vi "runner.vi"() -> ()   [LabVIEW 2010]
uses:
  common/xcontrols/XUserDropdown/XUserDropdown/XUserDropdown.xctl
  common/classes/ErrorController/ErrorController/ErrorController.lvclass
  <vilib>/Utility/miscctls.llb/LVPointTypeDef.ctl
  common/clusters/plugin_specification.ctl
  HelioWizardDL101109/wizard_cluster.ctl
  common/classes/GenericComponent/GenericComponent/GenericComponent.lvclass
  <vilib>/Platform/browser.llb/Open URL in Default Browser (string).vi
  common/classes/ErrorController/ErrorController/class_data.vi
panel:
  out "error loaded?":bool
  out "progress slider":i32(slide) scale=0.0..17.0
  in  "button: copy user":bool
  in  "button: delete user":bool
  in  "button: new user":bool
  in  "user":string(xcontrol)
  in  "mainConfigButton":bool
  in  "step":i32(listbox) caption="steps"
  in  "proceedButton":bool
  in  "backButton":bool
  in  "startButton":bool
  in  "wizard":string(combo) caption="Select a wizard"
  # "Wizard Runner"
  # "Procedure\n\n1. Select and start a wizard (it may take some time until all steps are loaded).\n\n2. Perform all configuration steps in the sequence given (note that there may be dependencies!).\n\n3. Edit main configuration.\n\nHint: Don't leave any component specifications empty in the configuration dialogs. Choose the generic version if a more specifiy component doesn't apply."
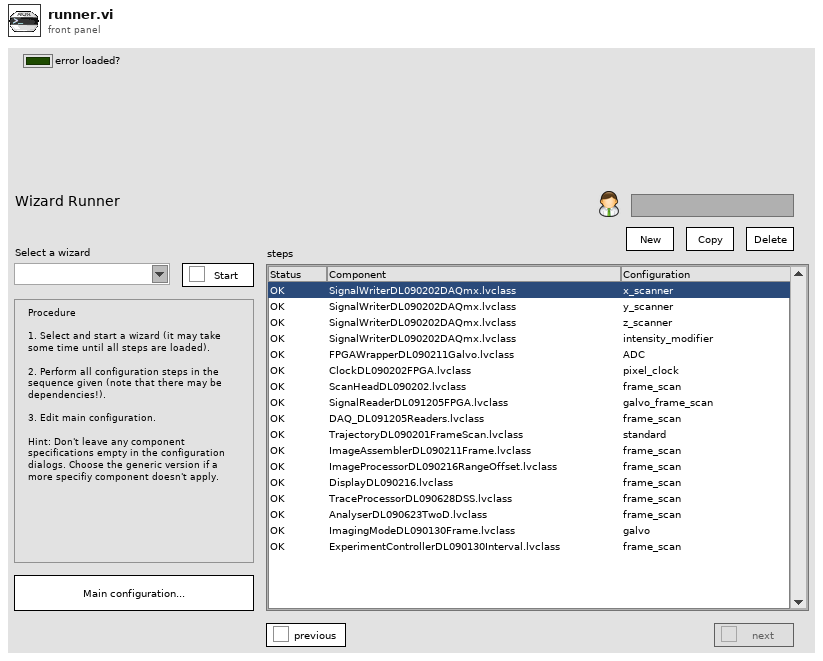
[diagram p1: front panel]
types:
  T1 = typedef "LVPointTypeDef.ctl" = cluster{"Horizontal":i16, "Vertical":i16}
  T2 = typedef "plugin_specification.ctl" = cluster{"class path":string, "configuration":string, "label":string, "settings name":string}
  T3 = typedef "wizard_cluster.ctl" = cluster{"step":T2[]}
  T4 = enum8{"Enabled", "Disabled", "Disabled and Grayed Out"}
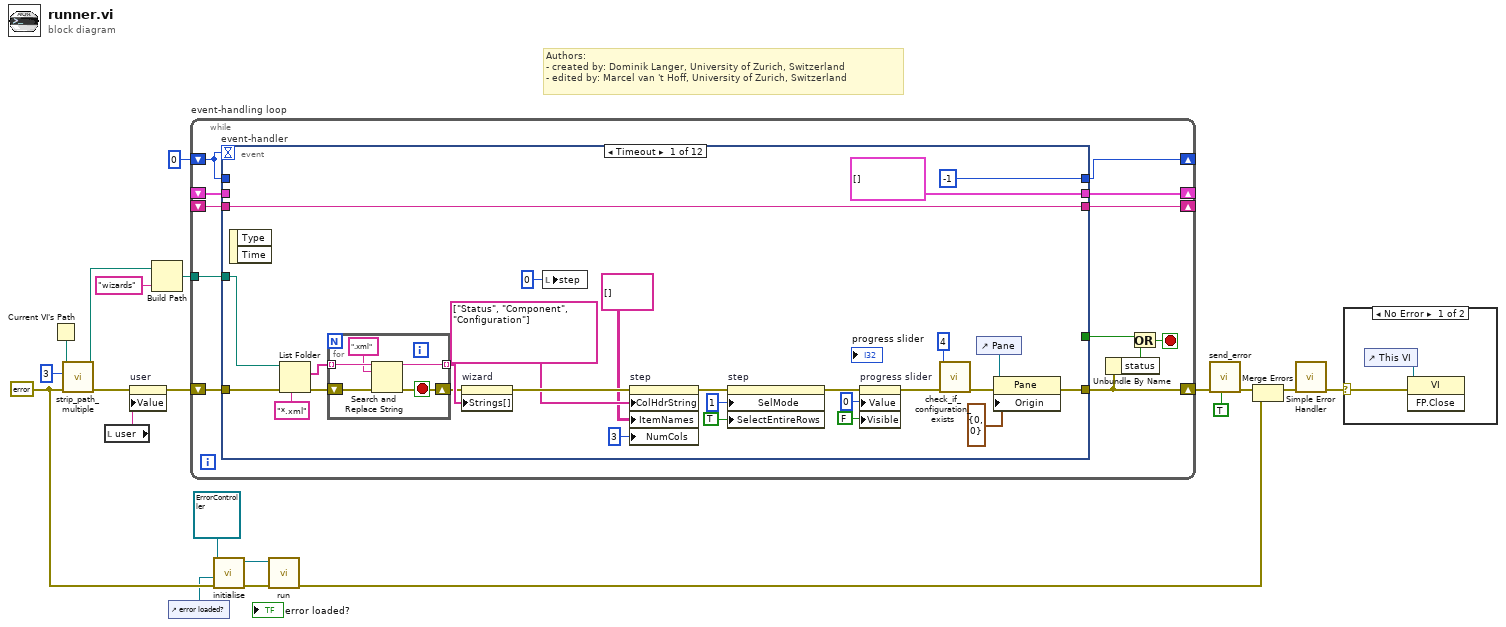
[diagram p0: block diagram]
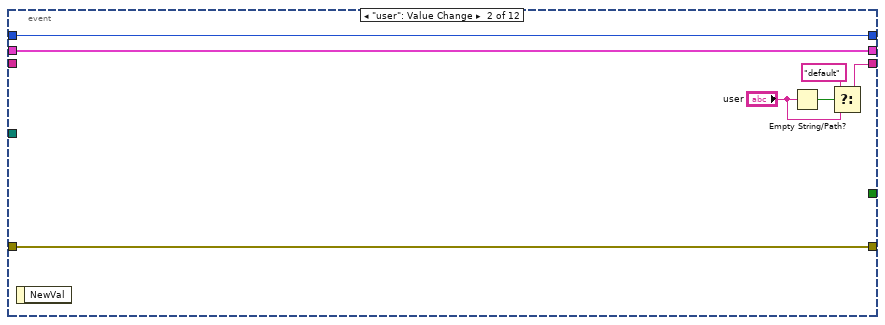
[diagram p3: hidden frame]
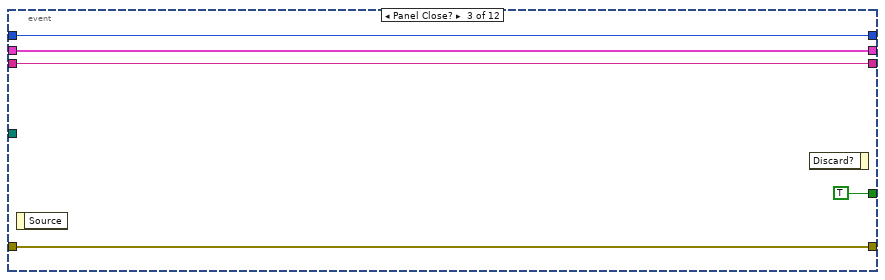
[diagram p4: hidden frame]
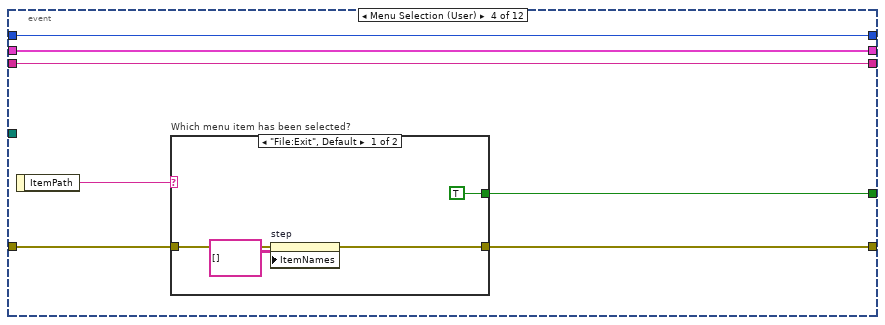
[diagram p5: hidden frame]
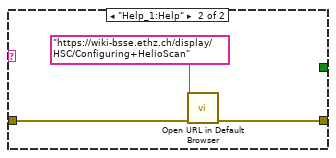
[diagram p6: hidden frame]
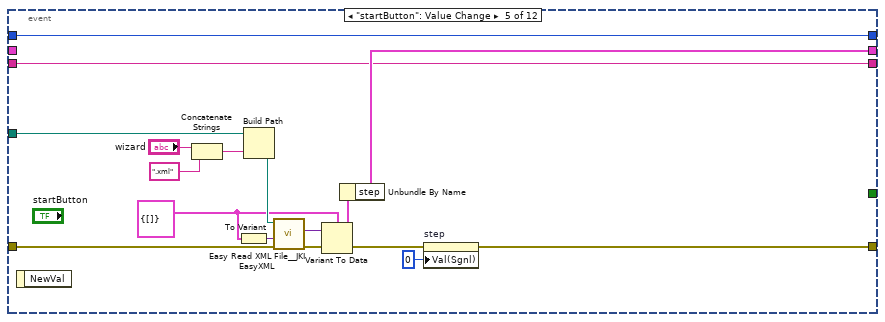
[diagram p7: hidden frame]
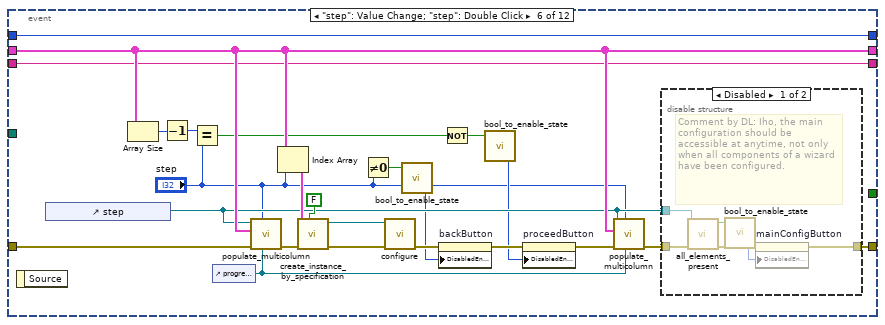
[diagram p8: hidden frame]
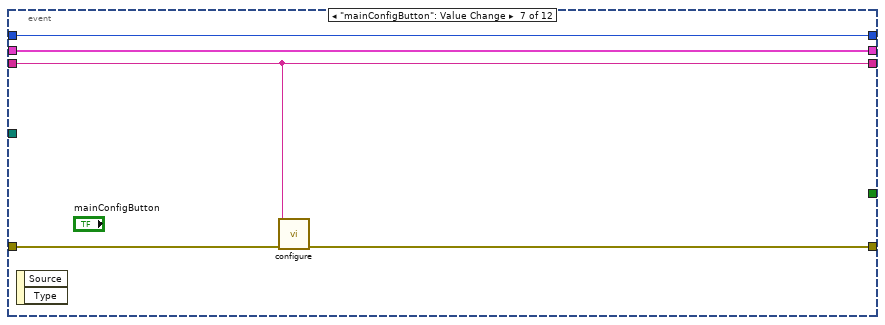
[diagram p10: hidden frame]
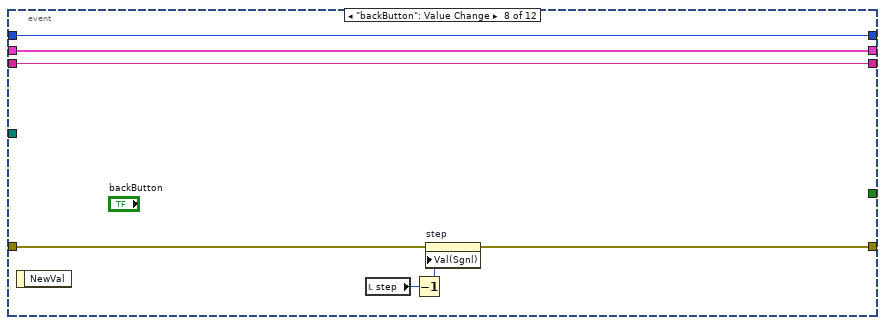
[diagram p11: hidden frame]
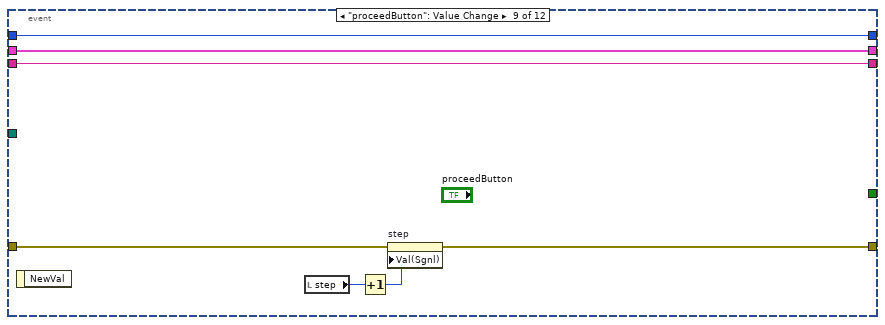
[diagram p12: hidden frame]
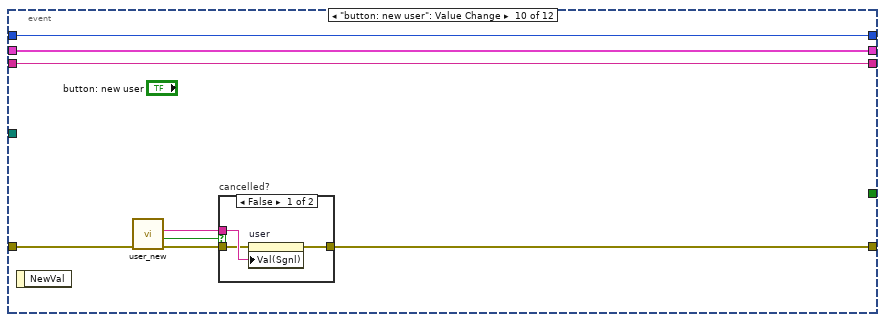
[diagram p13: hidden frame]
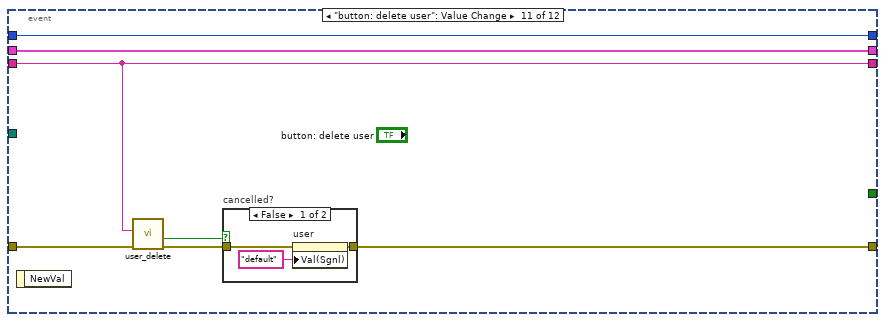
[diagram p15: hidden frame]
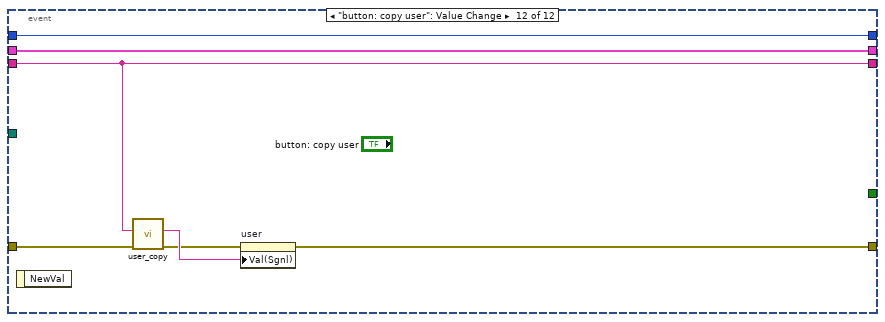
[diagram p17: hidden frame]
diagram:
  w5 = errorcluster {"status"=FALSE, "code"=0, "source"=""} ("error in (no error)")
  # "Authors: \n- created by: Dominik Langer, University of Zurich, Switzerland\n- edited by: Marcel van 't Hoff, University of Zurich, Switzerland"
  n1 = Current VI's Path() -> (path=w17:path)
  n2 = call "strip_path_multiple.vi"("error in (no error)"=w5, "number of strips"=3, "path in"=w17) -> ("error out"=w3:errorcluster, "path out"=w16:path)  [unwired: 7 in]
  n3 = local read "user"() -> (w1:string)
  n4 = property on="user" class="XUserDropdown (strict)"(error in=w3, "Value"=w1) -> (error out=w2:errorcluster)  [unwired: 1 in, 1 out]
  n5 = Build Path(base path=w16, name or relative path="wizards") -> (appended path=w18:path)
  n6 = control-ref of="error loaded?"() -> (w4:refnum<vi>)
  n7 = while "event-handling loop" {
    tunnel: w18 -> [w27]
    shift-right: [w25] -> _
    shift-left: _ -> [w26]
    shift-right: [w23] -> _
    shift-left: 0 -> [w24]
    shift-right: [w22] -> _
    shift-left: _ -> [w21]
    shift-right: [w31] -> w10
    shift-left: w2 -> [w32]
    stop <- w28 stop-if-true
    n8 = event "event-handler" shown="[0] Timeout" {
      selector: _ -> [_ _ _ _ _ _ _ _ _ _ _ _]
      dyn-events: _ -> [_ _ _ _ _ _ _ _ _ _ _ _]
      timeout: w24 -> [_ _ _ _ _ _ _ _ _ _ _ _]
      tunnel: w32 -> [w56 w69 w76 w79 w107 w124 w141 w145 w153 w162 w174 w185]
      tunnel: [w35 w69 w76 w78 w95 w118 w140 w148 w152 w159 w171 w181] -> w31
      tunnel: [_ _ TRUE w80 _ _ _ _ _ _ _ _] -> w29
      tunnel: w27 -> [w57 _ _ _ w106 _ _ _ _ _ _ _]
      tunnel: [T2[] [] w71 w74 w83 w98 w121 w143 w150 w157 w165 w176 w187] -> w25
      tunnel: w26 -> [_ w71 w74 w83 _ w121 w143 w150 w157 w165 w176 w187]
      tunnel: [-1 w70 w73 w82 w101 w126 w142 w149 w156 w164 w175 w186] -> w23
      tunnel: w24 -> [_ w70 w73 w82 w101 w126 w142 w149 w156 w164 w175 w186]
      tunnel: [w46 w66 w72 w77 w94 w117 w139 w144 w151 w163 w173 w184] -> w22
      tunnel: w21 -> [w46 _ w72 w77 w94 w117 w139 w144 w151 w163 w173 w184]
      event Timeout {
        n9 = event-data() -> ()  [unwired: 1 in, 2 out]
        n10 = List Folder(path=w57, pattern="*.xml", error in=w56) -> (filenames=w40:string[], error out=w38:errorcluster)  [unwired: 1 in, 2 out]
        n11 = for {
          tunnel: w40 -> [w64] mode=indexing
          tunnel: [w62] -> w39 mode=indexing
          shift-right: [w60] -> w37
          shift-left: w38 -> [w61]
          stop <- w60 stop-if-true
          n12 = Search and Replace String(input string=w64, search string=".xml", error in=w61) -> (result string=w62:string, error out=w60:errorcluster)  [unwired: 5 in, 2 out]
        }
        n13 = property on="wizard" class="CmbBox"(error in=w37, "Strings[]"=w39) -> (error out=w54:errorcluster)  [unwired: 1 in, 1 out]
        n14 = local write "step"(0 ("step")) -> ()
        n15 = property on="step" class="MCListbox (strict)"(error in=w54, "ColHdrString"=string[] ["Status", "Component", "Configuration"] ("Item Names"), "ItemNames"=string[][] [] ("Item Names"), "NumCols"=u32 3 ("Number of Columns")) -> (error out=w48:errorcluster)  [unwired: 1 in, 1 out]
        n16 = property on="step" class="MCListbox (strict)"(error in=w48, "SelMode"=1 ("Selection Mode"), "SelectEntireRows"=TRUE ("Select Entire Rows")) -> (error out=w43:errorcluster)  [unwired: 1 in, 1 out]
        n17 = property on="progress slider" class="Slide (strict)"(error in=w43, "Value"=0 ("progress slider"), "Visible"=FALSE) -> (error out=w42:errorcluster)  [unwired: 1 in, 1 out]
        n18 = call "check_if_configuration_exists.vi"("error in (no error)"=w42, "number of strips"=4) -> ("error out"=w36:errorcluster)  [unwired: 9 in]
        n19 = control-ref of="Pane"() -> (w34:refnum<vi>)
        n20 = property class="Pane"(reference=w34, error in=w36, "Origin"=T1 {"Horizontal"=0, "Vertical"=0}) -> (error out=w35:errorcluster)  [unwired: 1 out]
      }
      event "user": Value Change {
        n21 = event-data() -> ()  [unwired: 1 in, 1 out]
        n22 = Empty String/Path?(string/path="user") -> (empty?=w68:bool)
        n23 = Select(t="default", s=w68, f="user") -> (s? t:f=w66:string)
      }
      event Panel Close? {
        n24 = event-data() -> ()  [unwired: 1 in, 1 out]
        n25 = event-data() -> ()  [unwired: 2 in, 1 out]
      }
      event Menu Selection (User) {
        n26 = event-data() -> ("ItemPath"=w81:string)  [unwired: 1 in]
        n27 = case "Which menu item has been selected?" shown="\"File:Exit\", Default" w81 {
          tunnel: [TRUE _] -> w80
          tunnel: w79 -> [w86 w90]
          tunnel: [w84 w89] -> w78
          frame "File:Exit", Default {
            n28 = property on="step" class="MCListbox (strict)"(error in=w86, "ItemNames"=string[][] [] ("Item Names")) -> (error out=w84:errorcluster)  [unwired: 1 in, 1 out]
          }
          frame "Help_1:Help" {
            n29 = call-poly <vilib>:"Open URL in Default Browser.vi"("error in (no error)"=w90, "URL"="https://wiki-bsse.ethz.ch/display/HSC/Configuring+HelioScan") -> ("error out"=w89:errorcluster)  [unwired: 4 in, 1 out]
          }
        }
      }
      event "startButton": Value Change {
        w99 = T3 {"step"=[]}
        n30 = event-data() -> ()  [unwired: 1 in, 1 out]
        n31 = Concatenate Strings("wizard", ".xml" ("string")) -> (w91:string)
        n32 = To Variant(anything=w99) -> (Variant=w104:variant)
        n33 = Build Path(base path=w106, name or relative path=w91) -> (appended path=w105:path)
        n34 = call <vilib>:"Easy Read XML File__JKI EasyXML.vi"("error in (no error)"=w107, "LabVIEW Data (Type)"=w104, "XML File Path"=w105) -> ("error out"=w103:errorcluster, "LabVIEW Data"=w102:variant)  [unwired: 6 in, 1 out]
        n35 = Variant To Data(error in=w103, Variant=w102, type=w99) -> (error out=w96:errorcluster, data=w100:T3)
        n36 = Unbundle By Name(w100) -> ("step"=w98:T2[])
        n37 = property on="step" class="MCListbox (strict)"(error in=w96, "Val(Sgnl)"=0 ("Value (Signaling)")) -> (error out=w95:errorcluster)  [unwired: 1 in, 1 out]
      }
      event "step": Value Change; "step": Double Click {
        n38 = event-data() -> ()  [unwired: 1 in, 1 out]
        n39 = control-ref of="step"() -> (w119:refnum<vi>)
        n40 = Array Size(array=w121) -> (size(s)=w128:i32)
        n41 = Decrement(x=w128) -> (x-1=w127:i32)
        n42 = Equal?(x=w127, y="step") -> (x = y?=w113:bool)
        n43 = control-ref of="progress slider"() -> (w116:refnum<vi>)
        n44 = call "populate_multicolumn.vi"("progress slider"=w116, "selected item (index)"="step", "error in (no error)"=w124, "steps"=w121, "multicolumn list box"=w119) -> ("error out"=w123:errorcluster)  [unwired: 6 in]
        n45 = Index Array(array=w121, index="step") -> (element=w131:T2)
        n46 = call "create_instance_by_specification.vi"("call constructor?"=FALSE, "error in (no error)"=w123, "component specification"=w131) -> ("error out"=w114:errorcluster, "GenericPlugin out"=w115:refnum<class "GenericComponent.lvclass">)  [unwired: 6 in, 1 out]
        n47 = Not Equal To 0?(x="step") -> (x != 0?=w109:bool)
        n48 = call-dynamic "configure.vi"("error in (no error)"=w114, "GenericPlugin in"=w115) -> ("error out"=w130:errorcluster)  [unwired: 8 in, 1 out]
        n49 = call "bool_to_enable_state.vi"("boolean in"=w109) -> ("enabled status out"=w110:T4)  [unwired: 4 in]
        n50 = property on="backButton" class="Bool"(error in=w130, "DisabledEnum"=w110) -> (error out=w129:errorcluster)  [unwired: 1 in, 1 out]
        n51 = Not(x=w113) -> (.not. x?=w111:bool)
        n52 = call "bool_to_enable_state.vi"("boolean in"=w111) -> ("enabled status out"=w112:T4)  [unwired: 4 in]
        n53 = property on="proceedButton" class="Bool"(error in=w129, "DisabledEnum"=w112) -> (error out=w122:errorcluster)  [unwired: 1 in, 1 out]
        n54 = call "populate_multicolumn.vi"("progress slider"=w116, "selected item (index)"="step", "error in (no error)"=w122, "steps"=w121, "multicolumn list box"=w119) -> ("error out"=w120:errorcluster)  [unwired: 6 in]
        n55 = disable-structure shown="Disabled" {
          disable-tunnel: w120 -> [w137 w138]
          disable-tunnel: w119 -> [w136 _]
          disable-tunnel: [w134 w138] -> w118
          frame Disabled {
            # "Comment by DL: Iho, the main configuration should be accessible at anytime, not only when all components of a wizard have been configured."
            n56 = call "all_elements_present.vi"("error in (no error)"=w137, "multicolumn list box"=w136) -> ("error out"=w135:errorcluster, "all elements are present"=w133:bool)  [unwired: 8 in]
            n57 = call "bool_to_enable_state.vi"("boolean in"=w133) -> ("enabled status out"=w132:T4)  [unwired: 4 in]
            n58 = property on="mainConfigButton" class="Bool"(error in=w135, "DisabledEnum"=w132) -> (error out=w134:errorcluster)  [unwired: 1 in, 1 out]
          }
          frame Enabled {
          }
        }
      }
      event "mainConfigButton": Value Change {
        n59 = event-data() -> ()  [unwired: 1 in, 2 out]
        n60 = call "configure.vi"("error in (no error)"=w141, "user"=w139) -> ("error out"=w140:errorcluster)  [unwired: 8 in, 1 out]
      }
      event "backButton": Value Change {
        n61 = event-data() -> ()  [unwired: 1 in, 1 out]
        n62 = local read "step"() -> (w146:i32)
        n63 = Decrement(x=w146) -> (x-1=w147:i32)
        n64 = property on="step" class="MCListbox (strict)"(error in=w145, "Val(Sgnl)"=w147) -> (error out=w148:errorcluster)  [unwired: 1 in, 1 out]
      }
      event "proceedButton": Value Change {
        n65 = event-data() -> ()  [unwired: 1 in, 1 out]
        n66 = local read "step"() -> (w155:i32)
        n67 = Increment(x=w155) -> (x+1=w154:i32)
        n68 = property on="step" class="MCListbox (strict)"(error in=w153, "Val(Sgnl)"=w154) -> (error out=w152:errorcluster)  [unwired: 1 in, 1 out]
      }
      event "button: new user": Value Change {
        n69 = event-data() -> ()  [unwired: 1 in, 1 out]
        n70 = call "user_new.vi"("error in (no error)"=w162) -> ("error IO"=w160:errorcluster, "cancelled?"=w158:bool, "user name out"=w161:string)  [unwired: 8 in]
        n71 = case "cancelled?" shown="False" w158 {
          tunnel: w161 -> [w168 _]
          tunnel: w160 -> [w167 w169]
          tunnel: [w166 w169] -> w159
          frame False {
            n72 = property on="user" class="XUserDropdown (strict)"(error in=w167, "Val(Sgnl)"=w168) -> (error out=w166:errorcluster)  [unwired: 1 in, 1 out]
          }
          frame True {
          }
        }
      }
      event "button: delete user": Value Change {
        n73 = event-data() -> ()  [unwired: 1 in, 1 out]
        n74 = call "user_delete.vi"("error in (no error)"=w174, "user name in"=w173) -> ("error out"=w172:errorcluster, "cancelled?"=w170:bool)  [unwired: 8 in]
        n75 = case "cancelled?" shown="False" w170 {
          tunnel: w172 -> [w178 w180]
          tunnel: [w177 w180] -> w171
          frame False {
            n76 = property on="user" class="XUserDropdown (strict)"(error in=w178, "Val(Sgnl)"="default" ("Value (Signaling)")) -> (error out=w177:errorcluster)  [unwired: 1 in, 1 out]
          }
          frame True {
          }
        }
      }
      event "button: copy user": Value Change {
        n77 = event-data() -> ()  [unwired: 1 in, 1 out]
        n78 = call "user_copy.vi"("error in (no error)"=w185, "old user name in"=w184) -> ("error out"=w182:errorcluster, "new user name out"=w183:string)  [unwired: 7 in, 1 out]
        n79 = property on="user" class="XUserDropdown (strict)"(error in=w182, "Val(Sgnl)"=w183) -> (error out=w181:errorcluster)  [unwired: 1 in, 1 out]
      }
    }
    n80 = Unbundle By Name(w31) -> ("status"=w30:bool)
    n81 = Or(x=w29, y=w30) -> (x .or. y?=w28:bool)
  }
  n82 = call-dynamic "initialise.vi"("error in (no error)"=w5, "error boolean"=w4, "ErrorController in"=refnum<class "ErrorController.lvclass"> refnum) -> ("error out"=w12:errorcluster, "ErrorController out"=w11:refnum<class "ErrorController.lvclass">)  [unwired: 7 in]
  n83 = call "run.vi"("error in (no error)"=w12, "ErrorController in"=w11) -> ("error out"=w8:errorcluster)  [unwired: 8 in, 1 out]
  n84 = call "send_error.vi"("last error? (F)"=TRUE, "error in (no error)"=w10) -> ("error out"=w7:errorcluster)  [unwired: 9 in]
  n85 = Merge Errors(w7, w8) -> (w6:errorcluster)
  n86 = call <vilib>:"Simple Error Handler.vi"("error in (no error)"=w6) -> ("error out"=w14:errorcluster)  [unwired: 4 in, 4 out]
  n87 = case shown="No Error" w14 {
    selector: w14 -> [w189 _]
    frame No Error {
      n88 = control-ref of="This VI"() -> (w188:refnum<vi>)
      n89 = invoke class="VI" method="FP.Close"(reference=w188, error in=w189) -> ()  [unwired: 1 in, 3 out]
    }
    frame Error {
    }
  }
